vi "getRFDataArray.vi"(8 "error in (no error)":errorcluster, 11 "DDSOutput in":refnum<class "DDSOutput.lvclass">) -> (0 "error out":errorcluster, 2 "rfDataArray":cluster{dbl[][]}[](array[cluster]), 3 "DDSOutput out":refnum<class "DDSOutput.lvclass">)   [LabVIEW 2011, in "Hardware.lvlib" / "Channels.lvlib" / "DDSOutput.lvclass"]
uses:
  DDSOutput.lvclass
  DDSOutput.lvclass/DDSOutput.ctl
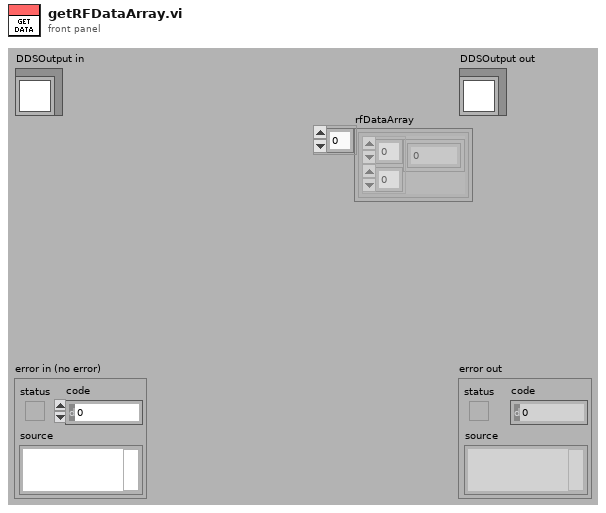
[diagram p1: front panel]
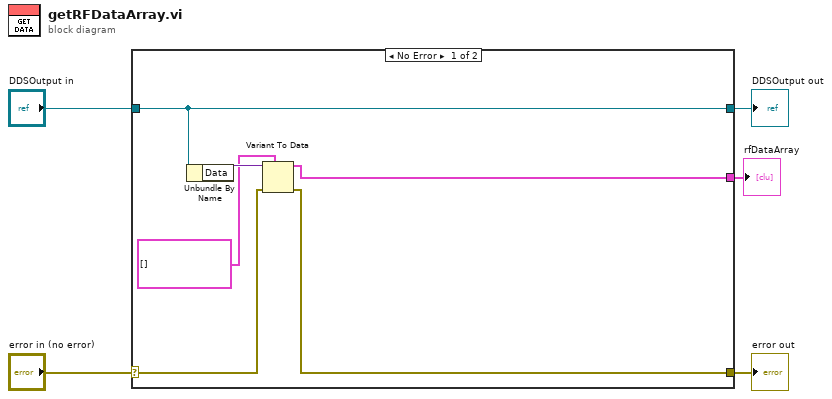
[diagram p0: block diagram]
diagram:
  n1 = case shown="No Error" "error in (no error)" {
    selector: "error in (no error)" -> [w9 w13]
    tunnel: [w7 w13] -> w4
    tunnel: [w11 w12] -> w2
    tunnel: "DDSOutput in" -> [w11 w12]
    tunnel: [w8 _] -> w1
    frame No Error {
      n2 = Unbundle By Name(w11) -> ("Data"=w10:variant)
      n3 = Variant To Data(error in=w9, type=cluster{dbl[][]}[] [], Variant=w10) -> (data=w8:cluster{dbl[][]}[], error out=w7:errorcluster)
    }
    frame Error {
    }
  }
  "error out" <- w4
  "DDSOutput out" <- w2
  "rfDataArray" <- w1
